vi "sree.vi"() -> ()   [LabVIEW 2025]
panel:
  out "x = LA":bool
  out "x = RE":bool
  out "x = RC":bool
  out "x = RF":bool
  out "x = RD":bool
  out "x = RA":bool
  out "x = LF":bool
  out "x =RB":bool
  out "x = LG":bool
  out "x = LD":bool
  out "x =LB":bool
  out "x = LE":bool
  out "x = LC":bool
  out "x = RG":bool
  in  "stop":bool
  out "text":string
  in  "file (use dialog)":path
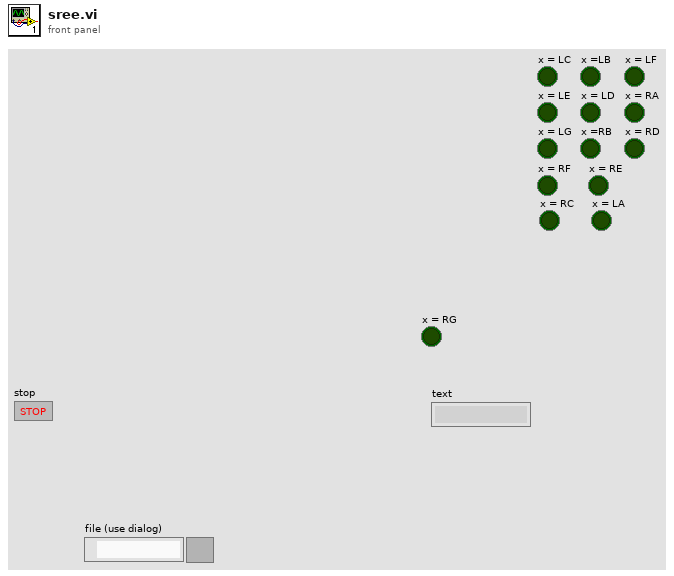
[diagram p1: front panel]
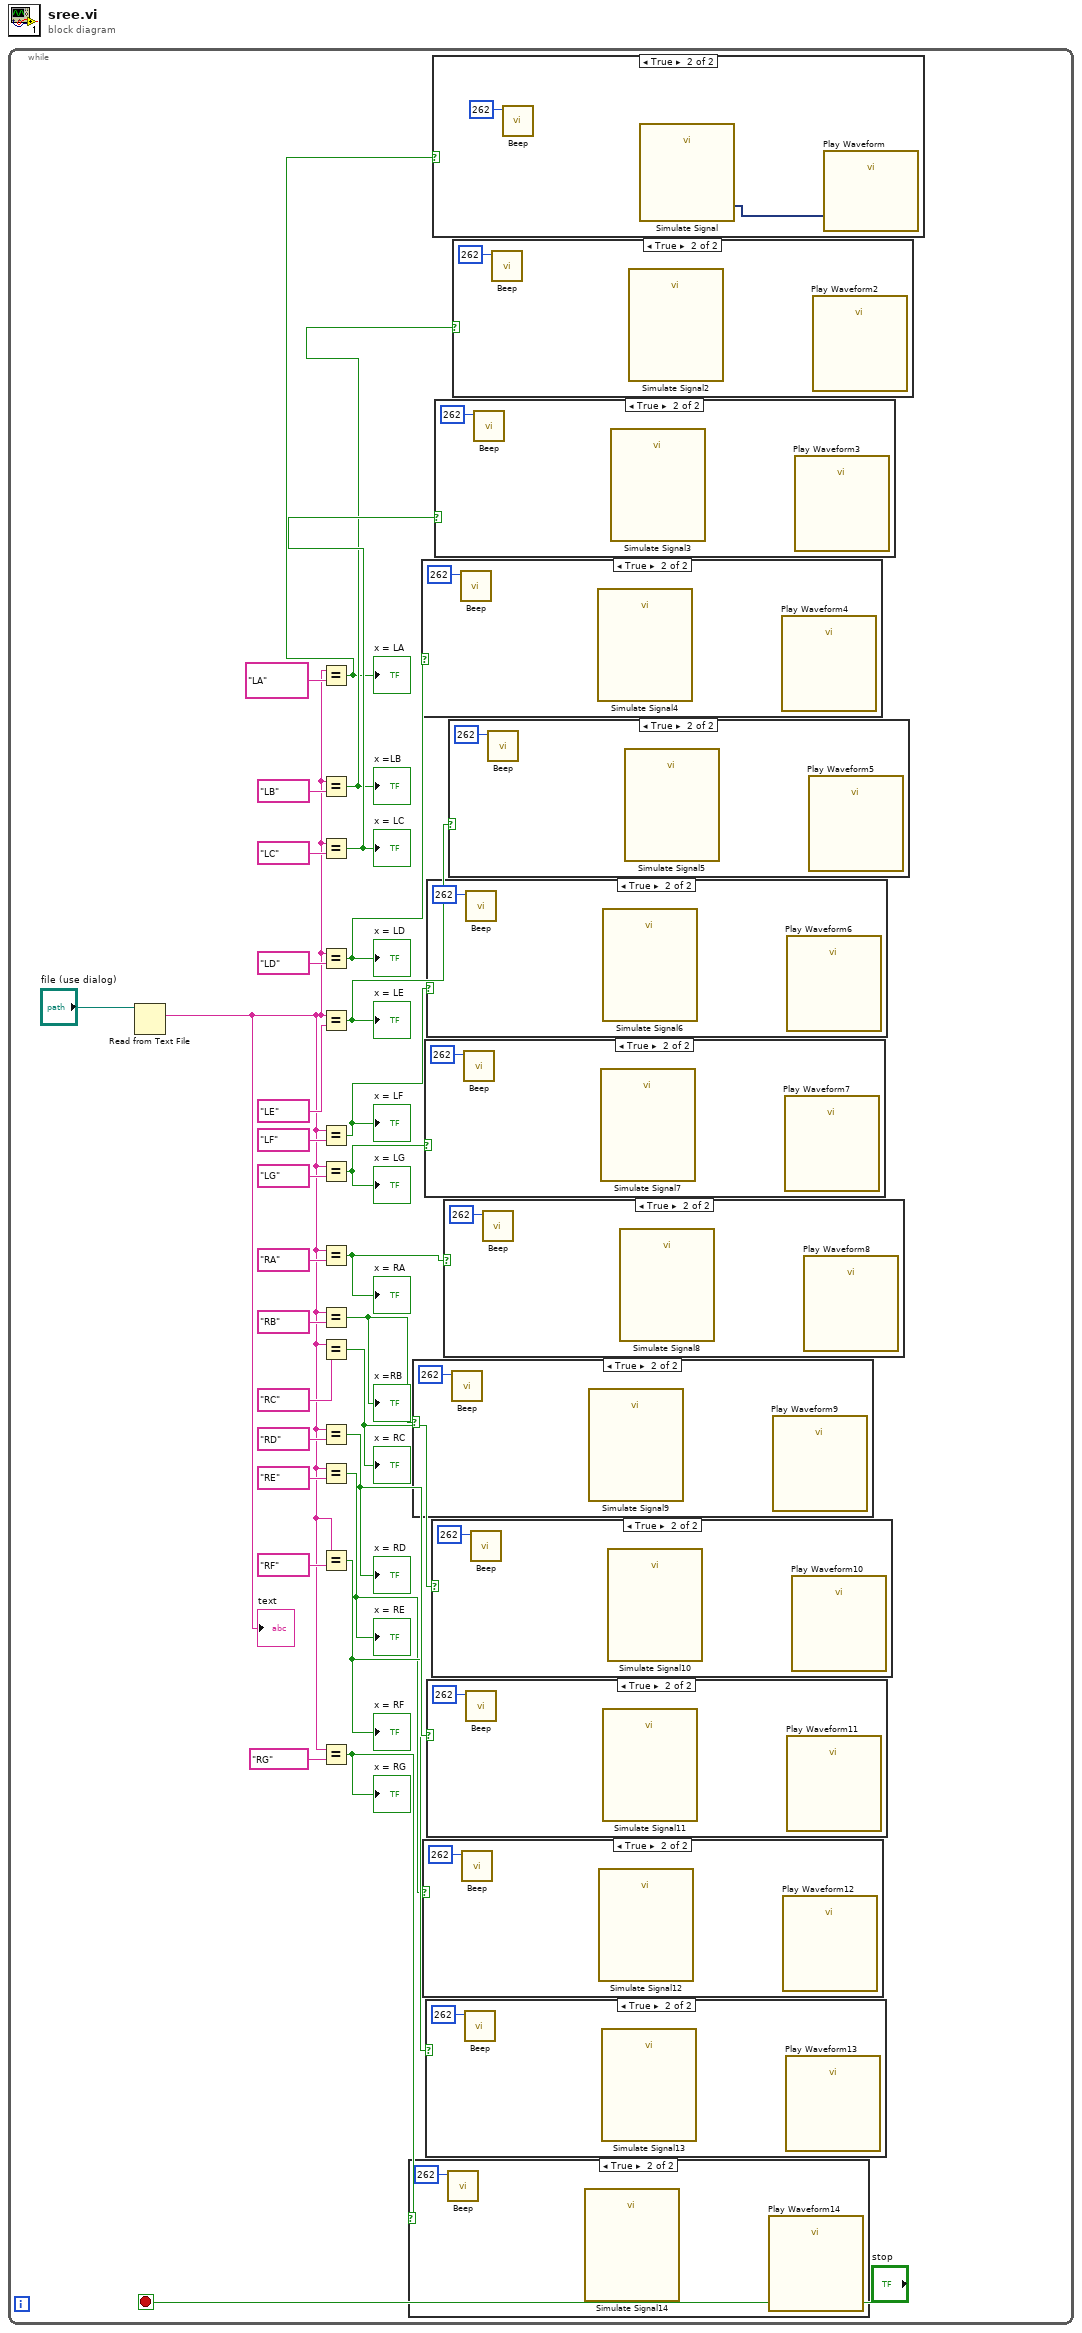
[diagram p0: block diagram]
diagram:
  n1 = while {
    stop <- "stop" stop-if-true
    n2 = Read from Text File(file (use dialog)="file (use dialog)") -> (text=w1:string)  [unwired: 3 in, 3 out]
    "text" <- w1
    n3 = Equal?(x=w1, y="LA") -> (x = y?=w2:bool)
    "x = LA" <- w2
    n4 = Equal?(x=w1, y="LB") -> (x = y?=w22:bool)
    "x =LB" <- w22
    n5 = Equal?(x=w1, y="LC") -> (x = y?=w26:bool)
    "x = LC" <- w26
    n6 = Equal?(x=w1, y="LD") -> (x = y?=w20:bool)
    "x = LD" <- w20
    n7 = Equal?(x=w1, y="LE") -> (x = y?=w24:bool)
    "x = LE" <- w24
    n8 = Equal?(x=w1, y="LF") -> (x = y?=w14:bool)
    "x = LF" <- w14
    n9 = Equal?(x=w1, y="LG") -> (x = y?=w18:bool)
    "x = LG" <- w18
    n10 = Equal?(x=w1, y="RA") -> (x = y?=w12:bool)
    "x = RA" <- w12
    n11 = Equal?(x=w1, y="RB") -> (x = y?=w16:bool)
    "x =RB" <- w16
    n12 = Equal?(x=w1, y="RC") -> (x = y?=w6:bool)
    "x = RC" <- w6
    n13 = Equal?(x=w1, y="RD") -> (x = y?=w10:bool)
    "x = RD" <- w10
    n14 = Equal?(x=w1, y="RE") -> (x = y?=w4:bool)
    "x = RE" <- w4
    n15 = Equal?(x=w1, y="RF") -> (x = y?=w8:bool)
    "x = RF" <- w8
    n16 = Equal?(x=w1, y="RG") -> (x = y?=w29:bool)
    "x = RG" <- w29
    n17 = case shown="True" w29 {
      frame False {
      }
      frame True {
        n18 = call <vilib>:"Beep.vi"("frequency (Hz)"=u32 262) -> ()  [unwired: 11 in]
        n19 = call "Simulate Signal14"() -> ()  [unwired: 14 in, 2 out]
        n20 = call "Play Waveform14"() -> ()  [unwired: 19 in, 1 out]
      }
    }
    n21 = case shown="True" w16 {
      frame False {
      }
      frame True {
        n22 = call <vilib>:"Beep.vi"("frequency (Hz)"=u32 262) -> ()  [unwired: 11 in]
        n23 = call "Simulate Signal9"() -> ()  [unwired: 14 in, 2 out]
        n24 = call "Play Waveform9"() -> ()  [unwired: 19 in, 1 out]
      }
    }
    n25 = case shown="True" w20 {
      frame False {
      }
      frame True {
        n26 = call <vilib>:"Beep.vi"("frequency (Hz)"=u32 262) -> ()  [unwired: 11 in]
        n27 = call "Simulate Signal4"() -> ()  [unwired: 14 in, 2 out]
        n28 = call "Play Waveform4"() -> ()  [unwired: 19 in, 1 out]
      }
    }
    n29 = case shown="True" w4 {
      frame False {
      }
      frame True {
        n30 = call <vilib>:"Beep.vi"("frequency (Hz)"=u32 262) -> ()  [unwired: 11 in]
        n31 = call "Simulate Signal12"() -> ()  [unwired: 14 in, 2 out]
        n32 = call "Play Waveform12"() -> ()  [unwired: 19 in, 1 out]
      }
    }
    n33 = case shown="True" w18 {
      frame False {
      }
      frame True {
        n34 = call <vilib>:"Beep.vi"("frequency (Hz)"=u32 262) -> ()  [unwired: 11 in]
        n35 = call "Simulate Signal7"() -> ()  [unwired: 14 in, 2 out]
        n36 = call "Play Waveform7"() -> ()  [unwired: 19 in, 1 out]
      }
    }
    n37 = case shown="True" w8 {
      frame False {
      }
      frame True {
        n38 = call <vilib>:"Beep.vi"("frequency (Hz)"=u32 262) -> ()  [unwired: 11 in]
        n39 = call "Simulate Signal13"() -> ()  [unwired: 14 in, 2 out]
        n40 = call "Play Waveform13"() -> ()  [unwired: 19 in, 1 out]
      }
    }
    n41 = case shown="True" w14 {
      frame False {
      }
      frame True {
        n42 = call <vilib>:"Beep.vi"("frequency (Hz)"=u32 262) -> ()  [unwired: 11 in]
        n43 = call "Simulate Signal6"() -> ()  [unwired: 14 in, 2 out]
        n44 = call "Play Waveform6"() -> ()  [unwired: 19 in, 1 out]
      }
    }
    n45 = case shown="True" w10 {
      frame False {
      }
      frame True {
        n46 = call <vilib>:"Beep.vi"("frequency (Hz)"=u32 262) -> ()  [unwired: 11 in]
        n47 = call "Simulate Signal11"() -> ()  [unwired: 14 in, 2 out]
        n48 = call "Play Waveform11"() -> ()  [unwired: 19 in, 1 out]
      }
    }
    n49 = case shown="True" w6 {
      frame False {
      }
      frame True {
        n50 = call <vilib>:"Beep.vi"("frequency (Hz)"=u32 262) -> ()  [unwired: 11 in]
        n51 = call "Simulate Signal10"() -> ()  [unwired: 14 in, 2 out]
        n52 = call "Play Waveform10"() -> ()  [unwired: 19 in, 1 out]
      }
    }
    n53 = case shown="True" w2 {
      frame False {
      }
      frame True {
        n54 = call <vilib>:"Beep.vi"("frequency (Hz)"=u32 262) -> ()  [unwired: 11 in]
        n55 = call "Simulate Signal"() -> ("Sine"=w32:dynamicdata)  [unwired: 14 in, 1 out]
        n56 = call "Play Waveform"("Data"=w32) -> ()  [unwired: 18 in, 1 out]
      }
    }
    n57 = case shown="True" w26 {
      frame False {
      }
      frame True {
        n58 = call <vilib>:"Beep.vi"("frequency (Hz)"=u32 262) -> ()  [unwired: 11 in]
        n59 = call "Simulate Signal3"() -> ()  [unwired: 14 in, 2 out]
        n60 = call "Play Waveform3"() -> ()  [unwired: 19 in, 1 out]
      }
    }
    n61 = case shown="True" w12 {
      frame False {
      }
      frame True {
        n62 = call <vilib>:"Beep.vi"("frequency (Hz)"=u32 262) -> ()  [unwired: 11 in]
        n63 = call "Simulate Signal8"() -> ()  [unwired: 14 in, 2 out]
        n64 = call "Play Waveform8"() -> ()  [unwired: 19 in, 1 out]
      }
    }
    n65 = case shown="True" w24 {
      frame False {
      }
      frame True {
        n66 = call <vilib>:"Beep.vi"("frequency (Hz)"=u32 262) -> ()  [unwired: 11 in]
        n67 = call "Simulate Signal5"() -> ()  [unwired: 14 in, 2 out]
        n68 = call "Play Waveform5"() -> ()  [unwired: 19 in, 1 out]
      }
    }
    n69 = case shown="True" w22 {
      frame False {
      }
      frame True {
        n70 = call <vilib>:"Beep.vi"("frequency (Hz)"=u32 262) -> ()  [unwired: 11 in]
        n71 = call "Simulate Signal2"() -> ()  [unwired: 14 in, 2 out]
        n72 = call "Play Waveform2"() -> ()  [unwired: 19 in, 1 out]
      }
    }
  }
